vi "Insert or Append or Replace.vi"(7 "Input Properties":T1={"Element Name (From JSON Path)"="U321", "Array Index"=0, "Array of Clusters?"=FALSE, "Element Present?"=TRUE, "Insert Element Key Name"="DBL", "Overwrite Data"=FALSE, "Process for 2D Array?"=FALSE}, 8 "error in (no error)":errorcluster, 9 "Functionality":T2(ring)=enum."Append", 10 "JSON Input Data Object":variant, 11 "JSON Upper Level":variant) -> (0 "error out":errorcluster, 1 "Functionality Applied":T2(ring), 3 "Modified Variant Out":variant)   [LabVIEW 2015]
uses:
  Type Definitions/Modify Variants TypeDef.ctl
  <vilib>/Utility/Data Type/NI_Data Type.lvlib
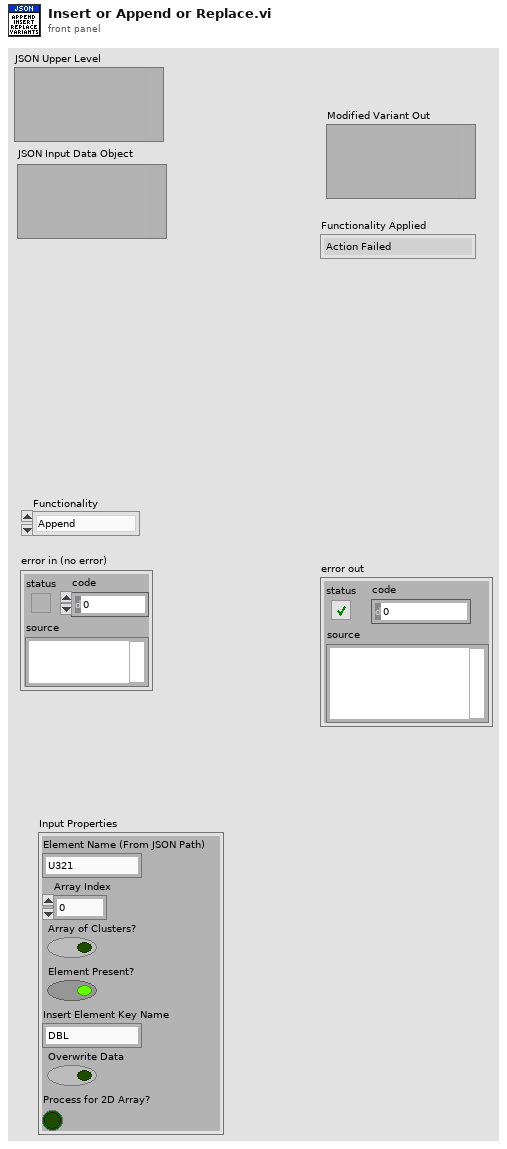
[diagram p1: front panel]
types:
  T1 = typedef "Modify Variants TypeDef.ctl" = cluster{"Element Name (From JSON Path)":string, "Array Index":i32, "Array of Clusters?":bool, "Element Present?":bool, "Insert Element Key Name":string, "Overwrite Data":bool, "Process for 2D Array?":bool}
  T2 = enum16{"Action Failed", "Append", "Insert", "Replace"}
  T3 = typedef "NI_Data Type.lvlib/Data Type.ctl" = enum8{"Invalid Type", "Void", "I8", "I16", "I32", "I64", "U8", "U16", "U32", "U64", "Single Float", "Double Float", "Extended Float", "Single Complex", "Double Complex", "Extended Complex", "Enum U8", "Enum U16", "Enum U32", "Enum U64", "Single Float With Unit", "Double Float With Unit", "Extended Float With Unit", "Single Complex with Unit", "Double Complex with Unit", "Extended Complex with Unit", "Boolean", "String", "Path", "Picture", "Tag", "Array", "Cluster", "Variant", "LV Variant", "Waveform", "Timestamp", "Digital Waveform", "Digital Data", "ExpressData", "Refnum", "External Data", "VI", "Poly VI", "LabVIEW Class Instance", "Fixed Point"}
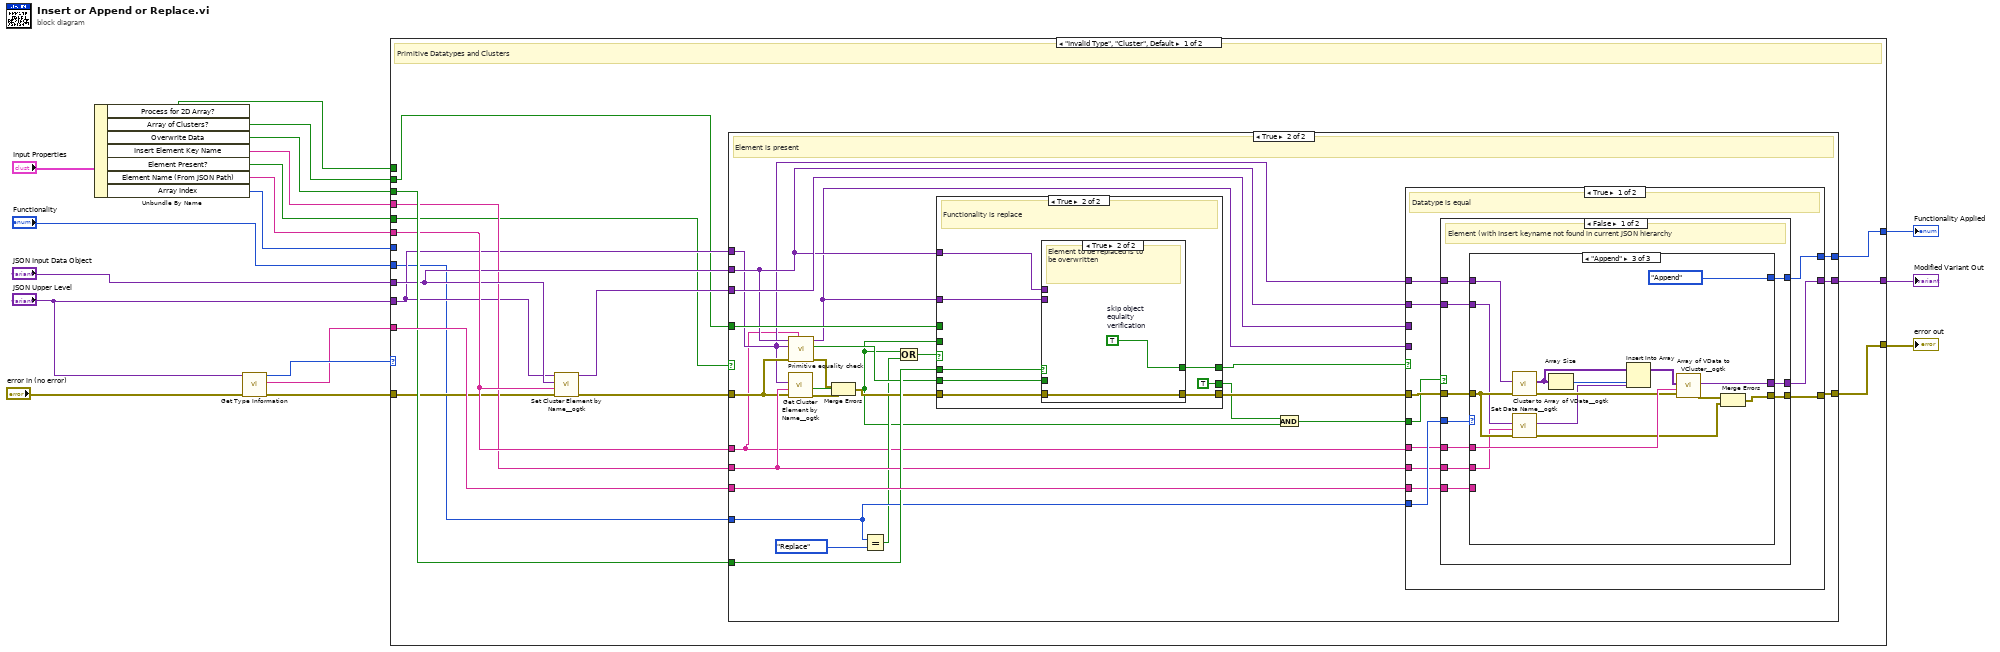
[diagram p0: block diagram]
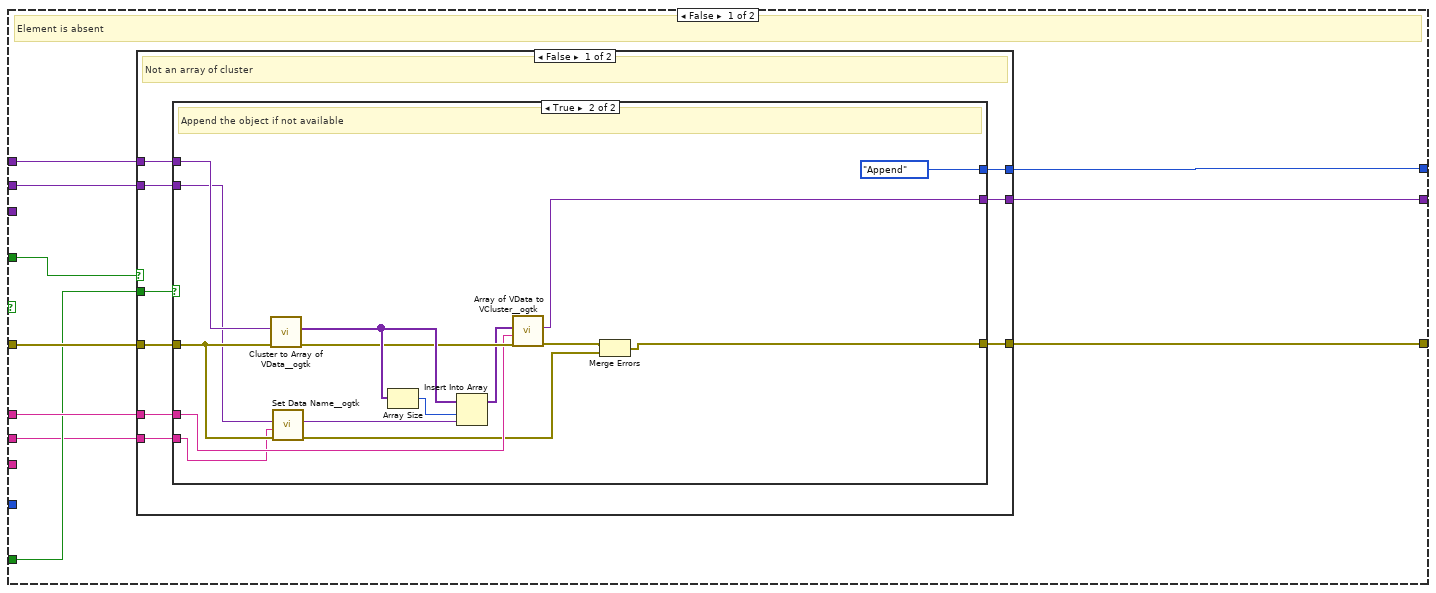
[diagram p2: hidden frame]
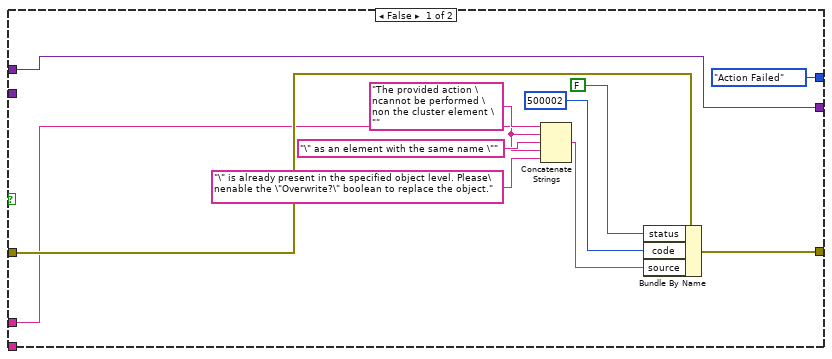
[diagram p3: hidden frame]
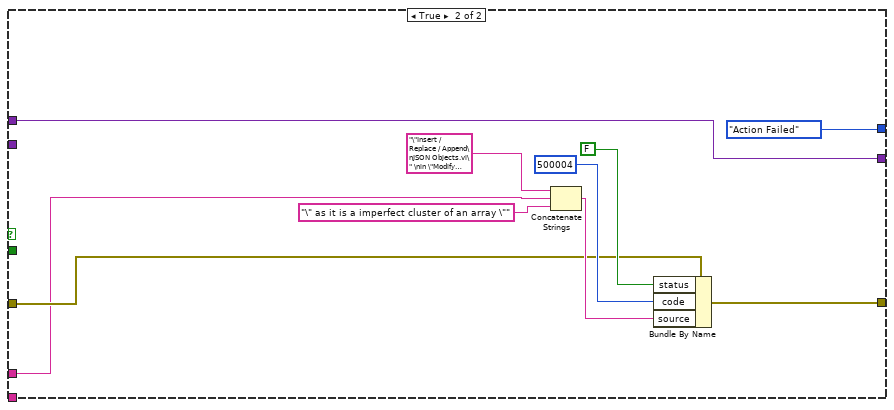
[diagram p4: hidden frame]
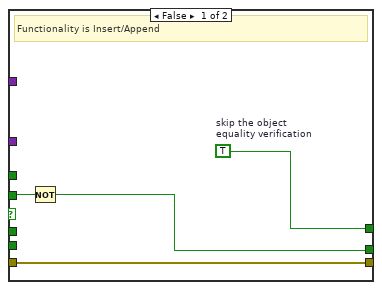
[diagram p5: hidden frame]
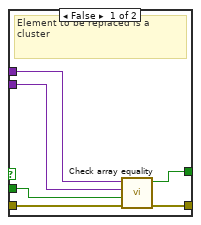
[diagram p6: hidden frame]
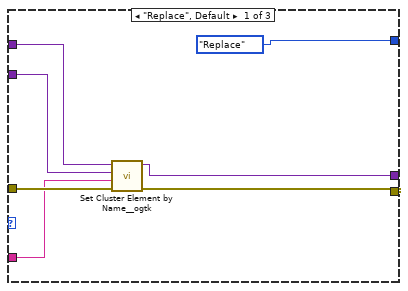
[diagram p7: hidden frame]
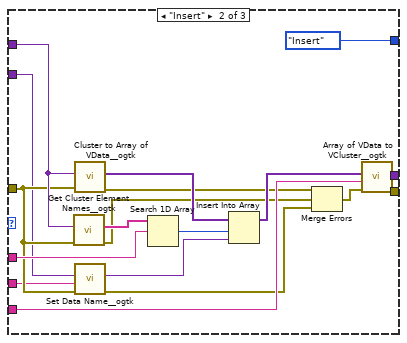
[diagram p8: hidden frame]
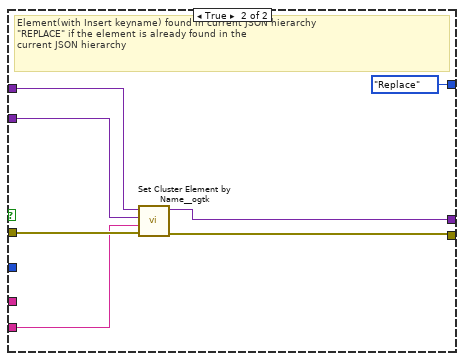
[diagram p9: hidden frame]
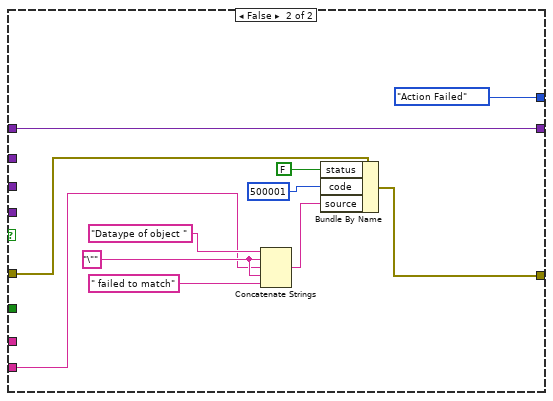
[diagram p10: hidden frame]
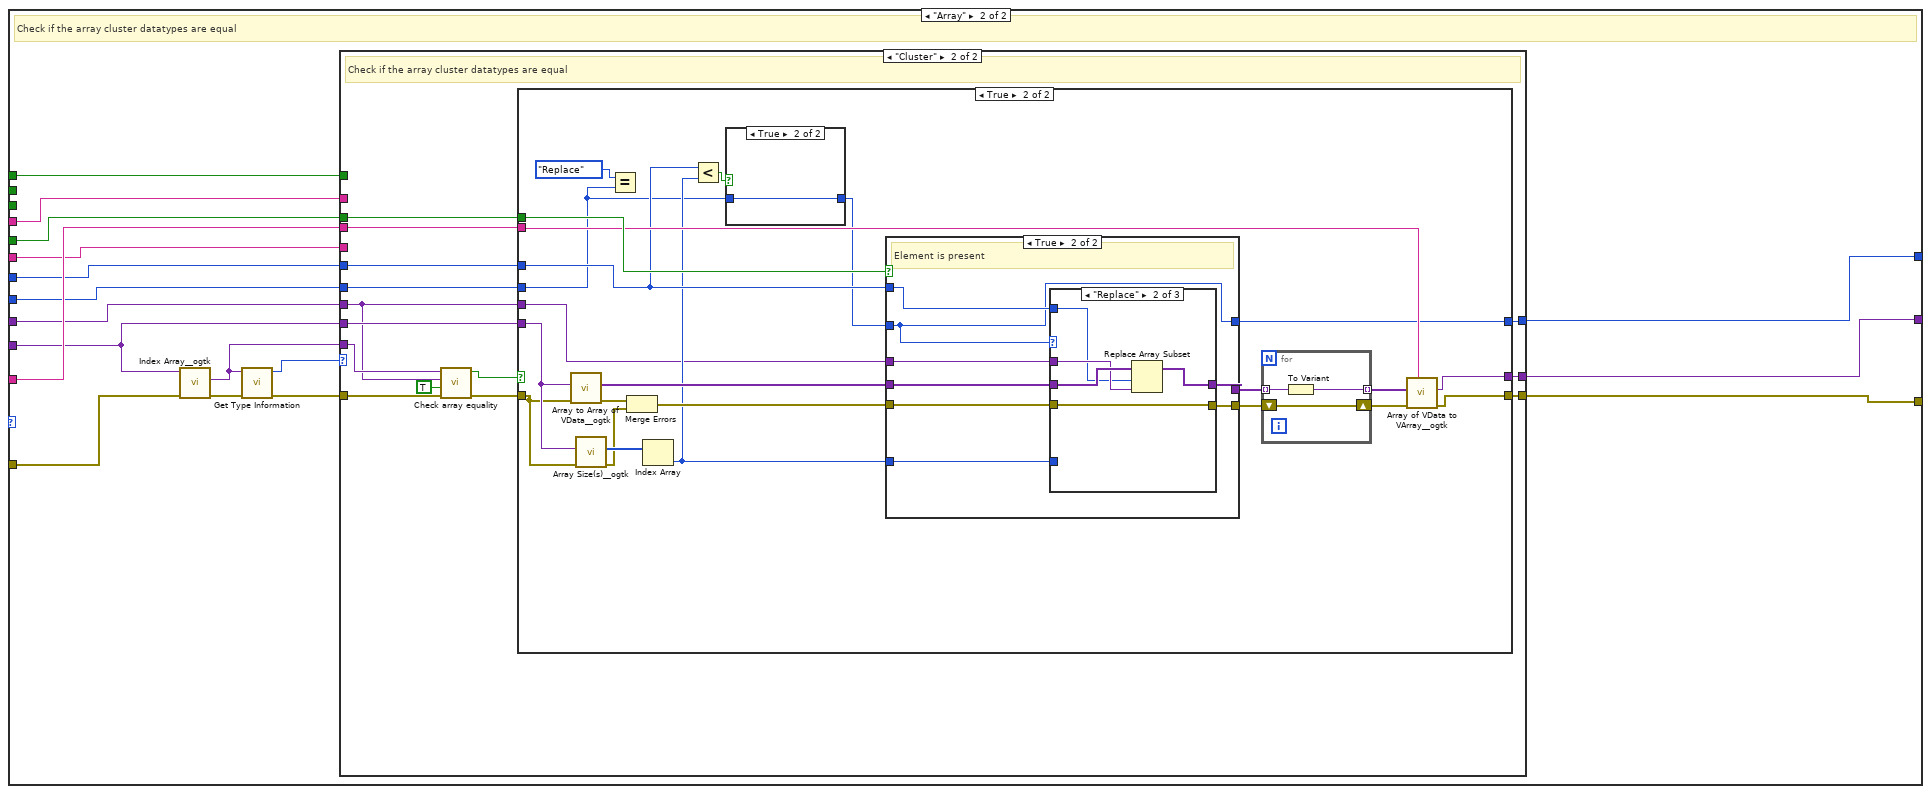
[diagram p11: hidden frame]
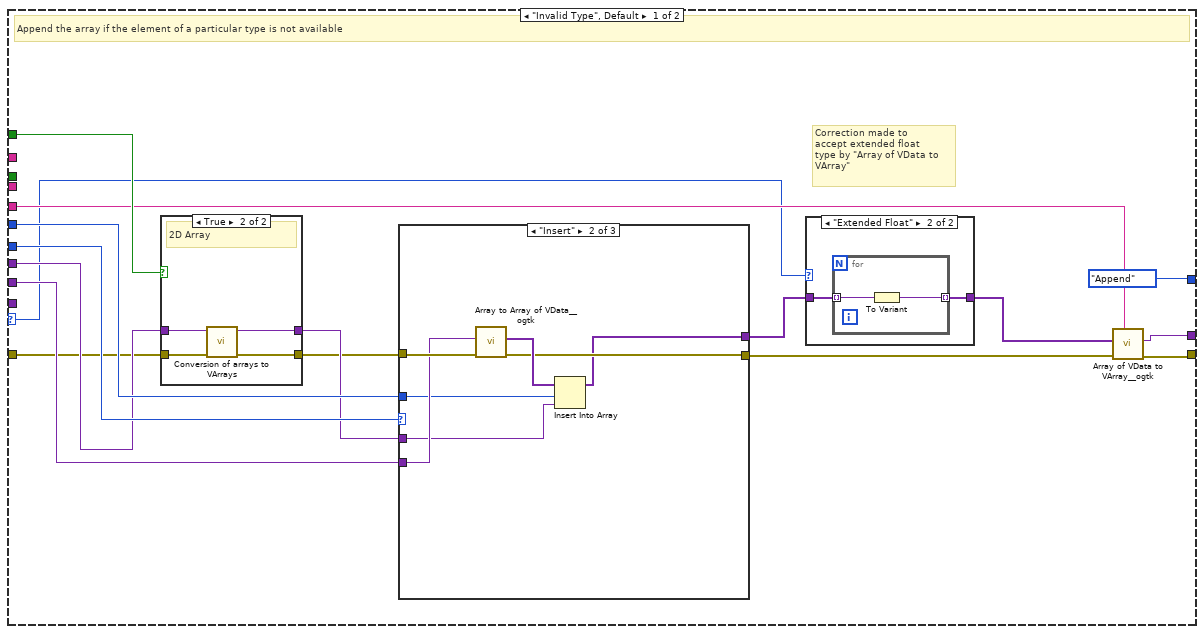
[diagram p12: hidden frame]
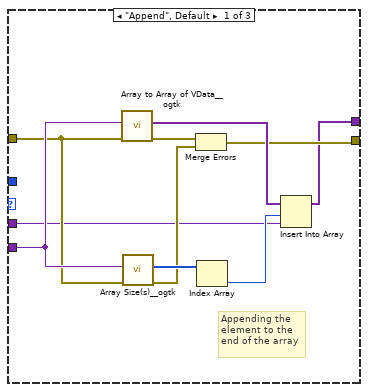
[diagram p15: hidden frame]
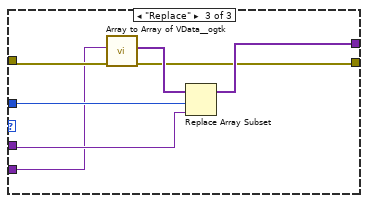
[diagram p16: hidden frame]
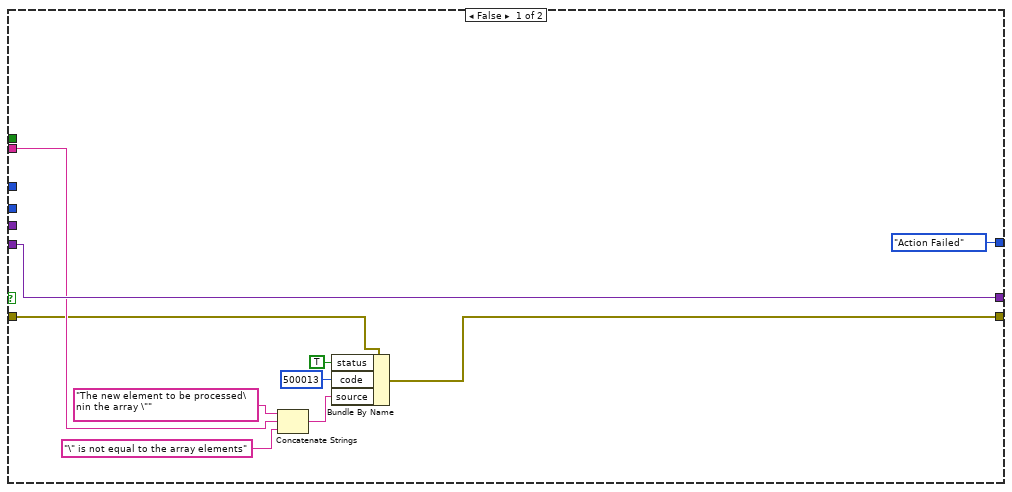
[diagram p17: hidden frame]
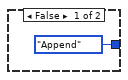
[diagram p18: hidden frame]
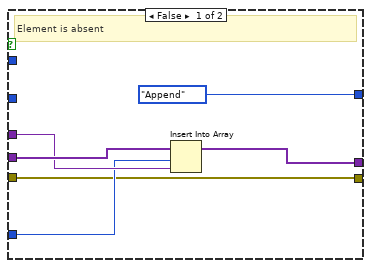
[diagram p19: hidden frame]
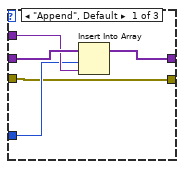
[diagram p20: hidden frame]
diagram:
  n1 = Unbundle By Name("Input Properties") -> ("Process for 2D Array?"=w1:bool, "Array of Clusters?"=w2:bool, "Overwrite Data"=w4:bool, "Insert Element Key Name"=w10:string, "Element Present?"=w14:bool, "Element Name (From JSON Path)"=w12:string, "Array Index"=w15:i32)
  n2 = call <vilib>:"Get Type Information.vi"("error in (no error)"="error in (no error)", "Variant"="JSON Upper Level") -> ("error out"=w5:errorcluster, "Name"=w6:string, "Type"=w7:T3)  [unwired: 5 in, 2 out]
  n3 = case shown="\"Invalid Type\", \"Cluster\", Default" w7 {
    tunnel: "JSON Upper Level" -> [w24 w222]
    tunnel: w5 -> [w23 w228]
    tunnel: [w32 w230] -> w17
    tunnel: w6 -> [w30 w229]
    tunnel: "JSON Input Data Object" -> [w26 w223]
    tunnel: "Functionality" -> [w22 w220]
    tunnel: w12 -> [w28 w216]
    tunnel: w15 -> [_ w221]
    tunnel: [w33 w219] -> w13
    tunnel: w14 -> [w20 w218]
    tunnel: [w31 w217] -> w16
    tunnel: w4 -> [w29 _]
    tunnel: w10 -> [w25 w215]
    tunnel: w2 -> [w21 _]
    tunnel: w1 -> [_ w214]
    frame "Invalid Type", "Cluster", Default {
      # "Primitive Datatypes and Clusters"
      n4 = call <userlib>:"Set Cluster Element by Name__ogtk.vi"("error in (no error)"=w23, "Element Name (\"\": New Element Data Name)"=w28, "New Element Value"=w26, "Cluster"=w24) -> ("error out"=w19:errorcluster, "VCluster out"=w27:variant)  [unwired: 5 in, 1 out]
      n5 = case shown="True" w20 {
        tunnel: [w43 w113] -> w33
        tunnel: [w41 w112] -> w32
        tunnel: w26 -> [w38 w99]
        tunnel: w19 -> [w42 w100]
        tunnel: [w36 w111] -> w31
        tunnel: w30 -> [_ w110]
        tunnel: w29 -> [w39 w107]
        tunnel: w28 -> [w40 w89]
        tunnel: w22 -> [_ w102]
        tunnel: w27 -> [_ w108]
        tunnel: w24 -> [w37 w98]
        tunnel: w25 -> [w35 w105]
        tunnel: w21 -> [w34 w104]
        frame False {
          # "Element is absent"
          n6 = case shown="False" w34 {
            tunnel: [w52 w80] -> w43
            tunnel: w42 -> [w51 w83]
            tunnel: [w50 w82] -> w41
            tunnel: w40 -> [w49 w81]
            tunnel: w39 -> [w48 _]
            tunnel: w38 -> [w47 _]
            tunnel: w37 -> [w46 w80]
            tunnel: [w45 T2."Action Failed" ("Functionality")] -> w36
            tunnel: w35 -> [w44 _]
            frame False {
              # "Not an array of cluster"
              n7 = case shown="True" w48 {
                tunnel: w47 -> [_ w69]
                tunnel: [w54 w73] -> w52
                tunnel: [w55 w64] -> w50
                tunnel: w51 -> [w63 w70]
                tunnel: w49 -> [w58 w74]
                tunnel: w46 -> [w54 w77]
                tunnel: [T2."Action Failed" ("Functionality") T2."Append" ("Functionality")] -> w45
                tunnel: w44 -> [_ w66]
                frame False {
                  n8 = Concatenate Strings("The provided action \ncannot be performed \non the cluster element \"" ("source"), w58, "\" as an element with the same name \"" ("string"), w58, "\" is already present in the specified object level. Please\nenable the \"Overwrite?\" boolean to replace the object." ("string")) -> (w56:string)
                  n9 = Bundle By Name(cluster=w63, "status"=FALSE, "code"=500002, "source"=w56) -> (w55:errorcluster)
                }
                frame True {
                  # "Append the object if not available"
                  n10 = call <userlib>:"Cluster to Array of VData__ogtk.vi"("error in (no error)"=w70, "Cluster"=w77) -> ("error out"=w76:errorcluster, "Array of VData"=w78:variant[])  [unwired: 8 in]
                  n11 = call <userlib>:"Set Data Name__ogtk.vi"("error in (no error)"=w70, "Data Name"=w66, "Data"=w69) -> ("error out"=w67:errorcluster, "Renamed Data"=w68:variant)  [unwired: 7 in]
                  n12 = Array Size(array=w78) -> (size(s)=w71:i32)
                  n13 = Insert Into Array(array=w78, index=w71, new element=w68) -> (w75:variant[])
                  n14 = call <userlib>:"Array of VData to VCluster__ogtk.vi"("error in (no error)"=w76, "Cluster Name"=w74, "Array"=w75) -> ("error out"=w65:errorcluster, "VCluster"=w73:variant)  [unwired: 7 in]
                  n15 = Merge Errors(w65, w67) -> (w64:errorcluster)
                }
              }
            }
            frame True {
              n16 = Concatenate Strings("\"Insert / Replace / Append\nJSON Objects.vi\" \nin \"Modify Variants.vi\"\nThe provided action \ncannot be performed \non the cluster element \"" ("source"), w81, "\" as it is a imperfect cluster of an array \"" ("string")) -> (w84:string)
              n17 = Bundle By Name(cluster=w83, "status"=FALSE, "code"=500004, "source"=w84) -> (w82:errorcluster)
            }
          }
        }
        frame True {
          # "Element is present"
          n18 = call <userlib>:"Get Cluster Element by Name__ogtk.vi"("error in (no error)"=w100, "Element Name"=w105, "Cluster"=w98) -> ("error out"=w96:errorcluster, "found?"=w91:bool)  [unwired: 6 in, 1 out]
          n19 = call "Primitive equality check.vi"("<Final element name on JSON path>"=w89, "error in (no error)"=w100, "<Upper cluster level>"=w98, "<New element to be processed>"=w99) -> ("error out"=w94:errorcluster, "Equal and clusters?"=w101:bool, "<Queried object from upper cluster level>"=w97:variant)  [unwired: 5 in]
          n20 = Merge Errors(w94, w96) -> (w95:errorcluster)
          n21 = Equal?(x=w102, y=T2."Replace") -> (x = y?=w93:bool)
          n22 = Or(x=w91, y=w93) -> (x .or. y?=w92:bool)
          n23 = case shown="True" w92 {
            tunnel: [w117 w126] -> w106
            tunnel: [w118 w125] -> w114
            tunnel: w99 -> [_ w124]
            tunnel: w95 -> [w117 w121]
            tunnel: w97 -> [_ w123]
            tunnel: w107 -> [_ w122]
            tunnel: w101 -> [_ w120]
            tunnel: w91 -> [w116 _]
            tunnel: w104 -> [_ _]
            tunnel: [w115 TRUE] -> w103
            frame False {
              w118 = TRUE  # skip the object equality verification
              # "Functionality is Insert/Append"
              n24 = Not(x=w116) -> (.not. x?=w115:bool)
            }
            frame True {
              # "Functionality is replace"
              n25 = case shown="True" w122 {
                tunnel: w124 -> [w130 _]
                tunnel: [w132 w133] -> w126
                tunnel: [w131 w134] -> w125
                tunnel: w123 -> [w129 _]
                tunnel: w121 -> [w128 w133]
                tunnel: w120 -> [w127 _]
                frame False {
                  # "Element to be replaced is a cluster"
                  n26 = call "Check array equality.vi"("error in (no error)"=w128, "Equal and clusters?"=w127, "Element to be inserted"=w129, "Upper Level Cluster Ele"=w130) -> ("error out"=w132:errorcluster, "Equal?"=w131:bool)  [unwired: 6 in]
                }
                frame True {
                  w134 = TRUE  # skip object equlaity  verification
                  # "Element to be replaced is to\nbe overwritten"
                }
              }
            }
          }
          n27 = And(x=w103, y=w91) -> (x .and. y?=w90:bool)
          n28 = case shown="True" w114 {
            tunnel: w98 -> [w144 w213]
            tunnel: w89 -> [w141 _]
            tunnel: w106 -> [w143 w212]
            tunnel: w102 -> [w145 _]
            tunnel: [w138 w207] -> w112
            tunnel: [w137 w213] -> w113
            tunnel: [w136 T2."Action Failed" ("Functionality")] -> w111
            tunnel: w110 -> [w139 _]
            tunnel: w105 -> [w140 w203]
            tunnel: w99 -> [w142 _]
            tunnel: w108 -> [_ _]
            tunnel: w97 -> [_ _]
            tunnel: w90 -> [w135 _]
            frame True {
              # "Datatype is equal"
              n29 = case shown="False" w135 {
                tunnel: w145 -> [w155 _]
                tunnel: w144 -> [w154 w200]
                tunnel: w143 -> [w153 w202]
                tunnel: w142 -> [w152 w199]
                tunnel: w141 -> [w151 _]
                tunnel: w140 -> [w150 w196]
                tunnel: w139 -> [w149 _]
                tunnel: [w148 w201] -> w138
                tunnel: [w147 w198] -> w137
                tunnel: [w146 T2."Replace" ("Functionality")] -> w136
                frame False {
                  # "Element (with Insert keyname not found in current JSON hierarchy"
                  n30 = case shown="\"Append\"" w155 {
                    tunnel: w154 -> [w161 w172 w195]
                    tunnel: w153 -> [w162 w171 w187]
                    tunnel: w152 -> [w160 w168 w185]
                    tunnel: w151 -> [w159 w179 w191]
                    tunnel: w150 -> [_ w169 w186]
                    tunnel: w149 -> [_ w170 _]
                    tunnel: [w158 w174 w182] -> w148
                    tunnel: [w157 w175 w189] -> w147
                    tunnel: [T2."Replace" ("Functionality") T2."Insert" ("Functionality") T2."Append" ("Functionality")] -> w146
                    frame "Replace", Default {
                      n31 = call <userlib>:"Set Cluster Element by Name__ogtk.vi"("error in (no error)"=w162, "Element Name (\"\": New Element Data Name)"=w159, "New Element Value"=w160, "Cluster"=w161) -> ("error out"=w158:errorcluster, "VCluster out"=w157:variant)  [unwired: 5 in, 1 out]
                    }
                    frame "Insert" {
                      # "Final Operation"
                      n32 = call <userlib>:"Get Cluster Element Names__ogtk.vi"("error in (no error)"=w171, "Cluster"=w172) -> ("error out"=w164:errorcluster, "Element Names"=w180:string[])  [unwired: 8 in]
                      n33 = call <userlib>:"Cluster to Array of VData__ogtk.vi"("error in (no error)"=w171, "Cluster"=w172) -> ("error out"=w166:errorcluster, "Array of VData"=w178:variant[])  [unwired: 8 in]
                      n34 = call <userlib>:"Set Data Name__ogtk.vi"("error in (no error)"=w171, "Data Name"=w169, "Data"=w168) -> ("error out"=w163:errorcluster, "Renamed Data"=w167:variant)  [unwired: 7 in]
                      n35 = Search 1D Array(1D array=w180, element=w179) -> (index of element=w177:i32)  [unwired: 1 in]
                      n36 = Insert Into Array(array=w178, index=w177, new element=w167) -> (w176:variant[])
                      n37 = Merge Errors(w166, w164, w163) -> (w165:errorcluster)
                      n38 = call <userlib>:"Array of VData to VCluster__ogtk.vi"("error in (no error)"=w165, "Cluster Name"=w170, "Array"=w176) -> ("error out"=w174:errorcluster, "VCluster"=w175:variant)  [unwired: 7 in]
                    }
                    frame "Append" {
                      n39 = call <userlib>:"Cluster to Array of VData__ogtk.vi"("error in (no error)"=w187, "Cluster"=w195) -> ("error out"=w190:errorcluster, "Array of VData"=w194:variant[])  [unwired: 8 in]
                      n40 = call <userlib>:"Set Data Name__ogtk.vi"("error in (no error)"=w187, "Data Name"=w186, "Data"=w185) -> ("error out"=w181:errorcluster, "Renamed Data"=w184:variant)  [unwired: 7 in]
                      n41 = Array Size(array=w194) -> (size(s)=w193:i32)
                      n42 = Insert Into Array(array=w194, index=w193, new element=w184) -> (w192:variant[])
                      n43 = call <userlib>:"Array of VData to VCluster__ogtk.vi"("error in (no error)"=w190, "Cluster Name"=w191, "Array"=w192) -> ("error out"=w183:errorcluster, "VCluster"=w189:variant)  [unwired: 7 in]
                      n44 = Merge Errors(w183, w181) -> (w182:errorcluster)
                    }
                  }
                }
                frame True {
                  # "Element(with Insert keyname) found in current JSON hierarchy\n\"REPLACE\" if the element is already found in the\ncurrent JSON hierarchy"
                  n45 = call <userlib>:"Set Cluster Element by Name__ogtk.vi"("error in (no error)"=w202, "Element Name (\"\": New Element Data Name)"=w196, "New Element Value"=w199, "Cluster"=w200) -> ("error out"=w201:errorcluster, "VCluster out"=w198:variant)  [unwired: 5 in, 1 out]
                }
              }
            }
            frame False {
              w204 = "\""
              n46 = Concatenate Strings("Dataype of object " ("source"), w204, w203, w204, " failed to match" ("string")) -> (w208:string)
              n47 = Bundle By Name(cluster=w212, "status"=FALSE, "code"=500001, "source"=w208) -> (w207:errorcluster)
            }
          }
        }
      }
    }
    frame "Array" {
      # "Check if the array cluster datatypes are equal"
      n48 = call <userlib>:"Index Array__ogtk.vi"("error in (no error)"=w228, "MultiD Array"=w222) -> ("error out"=w227:errorcluster, "Array Element"=w224:variant)  [unwired: 8 in]
      n49 = call <vilib>:"Get Type Information.vi"("error in (no error)"=w227, "Variant"=w224) -> ("error out"=w225:errorcluster, "Type"=w226:T3)  [unwired: 5 in, 3 out]
      n50 = case shown="\"Cluster\"" w226 {
        selector: w226 -> [w231 _]
        tunnel: w223 -> [w241 w284]
        tunnel: w225 -> [w240 w287]
        tunnel: [w236 w293] -> w230
        tunnel: w229 -> [_ w291]
        tunnel: w224 -> [_ w285]
        tunnel: w222 -> [w246 w295]
        tunnel: [w238 w294] -> w219
        tunnel: w221 -> [w243 w289]
        tunnel: w220 -> [w244 w288]
        tunnel: w218 -> [_ w292]
        tunnel: [T2."Append" ("Functionality") w290] -> w217
        tunnel: w216 -> [w237 _]
        tunnel: w215 -> [_ _]
        tunnel: w214 -> [w242 _]
        frame "Invalid Type", Default {
          # "Correction made to\naccept extended float\ntype by \"Array of VData to\nVArray\""
          # "Append the array if the element of a particular type is not available"
          n51 = case shown="True" w242 {
            tunnel: w241 -> [w252 w255]
            tunnel: w240 -> [w253 w257]
            tunnel: [w253 w256] -> w235
            tunnel: [w252 w254] -> w239
            frame False {
              # "Primtive Types"
            }
            frame True {
              # "2D Array"
              n52 = call "Conversion of arrays to VArrays.vi"("error in (no error)"=w257, "JSON Variant"=w255) -> ("error out"=w256:errorcluster, "VArray to \nbe inserted"=w254:variant)  [unwired: 8 in]
            }
          }
          n53 = case shown="\"Insert\"" w244 {
            tunnel: w246 -> [w267 w273 w277]
            tunnel: [w260 w269 w275] -> w233
            tunnel: [w258 w268 w276] -> w234
            tunnel: w239 -> [w259 w271 w278]
            tunnel: w235 -> [w263 w274 w280]
            tunnel: w243 -> [_ w270 w279]
            frame "Append", Default {
              # "Appending the \nelement to the\nend of the array"
              n54 = call <userlib>:"Array to Array of VData__ogtk.vi"("error in (no error)"=w263, "MultiD Array"=w267) -> ("error out"=w262:errorcluster, "1D Array of Variants"=w265:variant[])  [unwired: 8 in]
              n55 = call <userlib>:"Array Size(s)__ogtk.vi"("error in (no error)"=w263, "Array"=w267) -> ("error out"=w261:errorcluster, "Size(s)"=w266:u32[])  [unwired: 7 in, 1 out]
              n56 = Merge Errors(w262, w261) -> (w260:errorcluster)
              n57 = Index Array(array=w266) -> (element=w264:u32)  [unwired: 1 in]
              n58 = Insert Into Array(array=w265, index=w264, new element=w259) -> (w258:variant[])
            }
            frame "Insert" {
              n59 = call <userlib>:"Array to Array of VData__ogtk.vi"("error in (no error)"=w274, "MultiD Array"=w273) -> ("error out"=w269:errorcluster, "1D Array of Variants"=w272:variant[])  [unwired: 8 in]
              n60 = Insert Into Array(array=w272, index=w270, new element=w271) -> (w268:variant[])
            }
            frame "Replace" {
              n61 = call <userlib>:"Array to Array of VData__ogtk.vi"("error in (no error)"=w280, "MultiD Array"=w277) -> ("error out"=w275:errorcluster, "1D Array of Variants"=w281:variant[])  [unwired: 8 in]
              n62 = Replace Array Subset(array=w281, new element=w278, index=w279) -> (w276:variant[])
            }
          }
          n63 = case shown="\"Extended Float\"" w231 {
            tunnel: w234 -> [w247 w249]
            tunnel: [w247 w248] -> w232
            frame "Invalid Type", Default {
            }
            frame "Extended Float" {
              n64 = for {
                tunnel: w249 -> [w251] mode=indexing
                tunnel: [w250] -> w248 mode=indexing
                n65 = To Variant(anything=w251) -> (Variant=w250:variant)
              }
            }
          }
          n66 = call <userlib>:"Array of VData to VArray__ogtk.vi"("Array Name"=w237, "error in (no error)"=w233, "1D Array of VData"=w232) -> ("error out"=w236:errorcluster, "VArray"=w238:variant)  [unwired: 7 in]
        }
        frame "Cluster" {
          # "Check if the array cluster datatypes are equal"
          n67 = call "Check array equality.vi"("error in (no error)"=w287, "Equal and clusters?"=TRUE ("Clusters?"), "Element to be inserted"=w284, "Upper Level Cluster Ele"=w285) -> ("error out"=w286:errorcluster, "Equal?"=w282:bool)  [unwired: 6 in]
          n68 = case shown="True" w282 {
            tunnel: w295 -> [w305 w328]
            tunnel: [w305 w327] -> w294
            tunnel: [w296 w326] -> w293
            tunnel: w292 -> [_ w325]
            tunnel: w291 -> [w300 w324]
            tunnel: [T2."Action Failed" ("Functionality") w323] -> w290
            tunnel: w289 -> [_ w312]
            tunnel: w288 -> [_ w310]
            tunnel: w286 -> [w297 w307]
            tunnel: w284 -> [_ w306]
            frame False {
              n69 = Concatenate Strings("The new element to be processed\nin the array \"" ("source"), w300, "\" is not equal to the array elements" ("string")) -> (w298:string)
              n70 = Bundle By Name(cluster=w297, "status"=TRUE, "code"=500013, "source"=w298) -> (w296:errorcluster)
            }
            frame True {
              n71 = call <userlib>:"Array to Array of VData__ogtk.vi"("error in (no error)"=w307, "MultiD Array"=w328) -> ("error out"=w319:errorcluster, "1D Array of Variants"=w322:variant[])  [unwired: 8 in]
              n72 = call <userlib>:"Array Size(s)__ogtk.vi"("error in (no error)"=w307, "Array"=w328) -> ("error out"=w320:errorcluster, "Size(s)"=w321:u32[])  [unwired: 7 in, 1 out]
              n73 = Equal?(x=T2."Replace" ("y"), y=w310) -> ()  [unwired: 1 out]
              n74 = Merge Errors(w319, w320) -> (w318:errorcluster)
              n75 = Index Array(array=w321) -> (element=w311:u32)  [unwired: 1 in]
              n76 = Less?(x=w312, y=w311) -> (x < y?=w309:bool)
              n77 = case shown="True" w309 {
                tunnel: w310 -> [_ w330]
                tunnel: [T2."Append" ("Functionality") w330] -> w308
                frame False {
                }
                frame True {
                }
              }
              n78 = case shown="True" w325 {
                tunnel: w306 -> [w338 w347]
                tunnel: w322 -> [w339 w346]
                tunnel: [w337 w345] -> w317
                tunnel: w308 -> [_ w342]
                tunnel: w312 -> [_ w344]
                tunnel: w311 -> [w336 w343]
                tunnel: [T2."Append" ("Functionality") w342] -> w323
                tunnel: w318 -> [w334 w341]
                tunnel: [w334 w340] -> w314
                frame False {
                  # "Element is absent"
                  n79 = Insert Into Array(array=w339, index=w336, new element=w338) -> (w337:variant[])
                }
                frame True {
                  # "Element is present"
                  n80 = case shown="\"Replace\"" w342 {
                    tunnel: w347 -> [w351 w356 w362]
                    tunnel: w346 -> [w352 w357 w361]
                    tunnel: [w350 w355 w360] -> w345
                    tunnel: w344 -> [_ w354 w359]
                    tunnel: w343 -> [w349 _ _]
                    tunnel: w341 -> [w348 w353 w358]
                    tunnel: [w348 w353 w358] -> w340
                    frame "Append", Default {
                      n81 = Insert Into Array(array=w352, index=w349, new element=w351) -> (w350:variant[])
                    }
                    frame "Replace" {
                      n82 = Replace Array Subset(array=w357, new element=w356, index=w354) -> (w355:variant[])
                    }
                    frame "Insert" {
                      n83 = Insert Into Array(array=w361, index=w359, new element=w362) -> (w360:variant[])
                    }
                  }
                }
              }
              n84 = for {
                tunnel: w317 -> [w333] mode=indexing
                tunnel: [w332] -> w316 mode=indexing
                shift-right: [w331] -> w315
                shift-left: w314 -> [w331]
                n85 = To Variant(anything=w333) -> (Variant=w332:variant)
              }
              n86 = call <userlib>:"Array of VData to VArray__ogtk.vi"("Array Name"=w324, "error in (no error)"=w315, "1D Array of VData"=w316) -> ("error out"=w326:errorcluster, "VArray"=w327:variant)  [unwired: 7 in]
            }
          }
        }
      }
    }
  }
  "error out" <- w17
  "Functionality Applied" <- w16
  "Modified Variant Out" <- w13
